vi "S2C_ExeScriptAbort.vi"(8 "Error In":errorcluster, 11 "Q-Ref":refnum<queue>) -> (0 "Error Out":errorcluster)   [LabVIEW 2015]
doc: "Changes the testing status to Aborted and calls the results case."
uses:
  Controls/S2C_ResultStatus.ctl
  Controls/S2C_ExePause.ctl
  Globals/S2C_Globals.vi
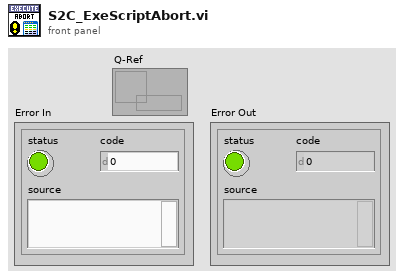
[diagram p1: front panel]
types:
  T1 = typedef "S2C_ExePause.ctl" = bool
  T2 = typedef "S2C_ResultStatus.ctl" = enum16{"Passed", "Failed", "Logged", "Aborted", "Error", "Testing...", "Paused", "No Record"}
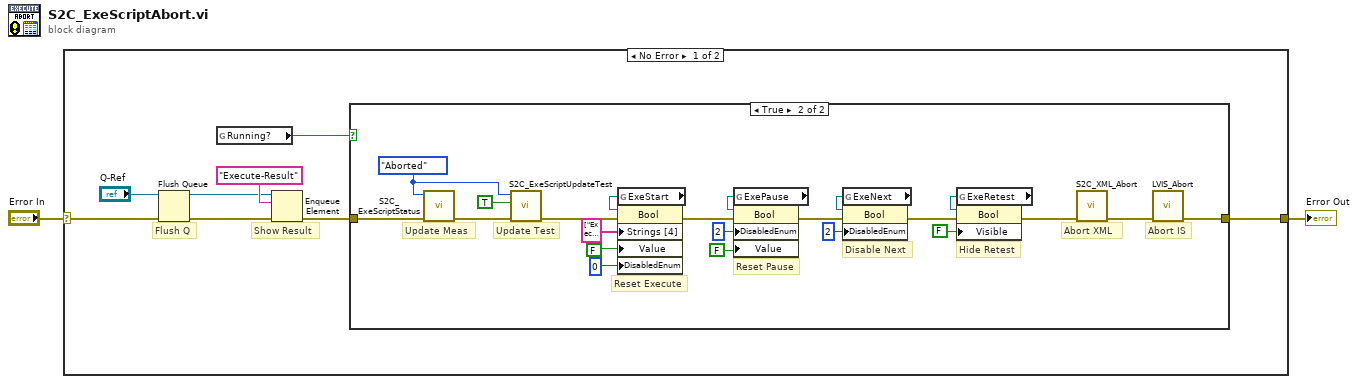
[diagram p0: block diagram]
diagram:
  n1 = case shown="No Error" "Error In" {
    selector: "Error In" -> [w8 w34]
    tunnel: [w7 w34] -> w1
    frame No Error {
      # "Show Result"
      # "Flush Q"
      n2 = Flush Queue(queue="Q-Ref", error in (no error)=w8) -> (queue out=w5:refnum<queue>, error out=w4:errorcluster)  [unwired: 1 out]
      n3 = global read "S2C_Globals.vi" "Running?"() -> (w10:bool)
      n4 = Enqueue Element(queue=w5, element="Execute-Result", error in (no error)=w4) -> (error out=w3:errorcluster)  [unwired: 1 in, 2 out]
      n5 = case shown="True" w10 {
        tunnel: [w11 w26] -> w7
        tunnel: w3 -> [w11 w33]
        frame False {
        }
        frame True {
          w18 = S2C_ResultStatus."Aborted" ("Status")
          # "Hide Retest"
          # "Update Test"
          # "Abort XML"
          # "Reset Execute"
          # "Abort IS"
          # "Disable Next"
          # "Reset Pause"
          # "Update Meas"
          n6 = call "S2C_ExeScriptStatus.vi"("Error In"=w33, "Status"=w18) -> ("Error Out"=w19:errorcluster)  [unwired: 9 in]
          n7 = call "S2C_ExeScriptUpdateTest.vi"("Error In"=w19, "LastMeas?"=TRUE, "Status"=w18) -> ("Error Out"=w17:errorcluster)  [unwired: 8 in]
          n8 = global read "S2C_Globals.vi" "ExeStart"() -> (w25:refnum<vi>)
          n9 = property on="Property Node" class="Bool"(reference=w25, error in=w17, "Strings [4]"=string[] ["Execute Script", "Abort Testing"] ("Array - String"), "Value"=T1 FALSE, "DisabledEnum"=u8 0) -> (error out=w22:errorcluster)  [unwired: 1 out]
          n10 = global read "S2C_Globals.vi" "ExePause"() -> (w32:refnum<vi>)
          n11 = property on="Property Node" class="Bool"(reference=w32, error in=w22, "DisabledEnum"=u8 2, "Value"=T1 FALSE) -> (error out=w28:errorcluster)  [unwired: 1 out]
          n12 = global read "S2C_Globals.vi" "ExeNext"() -> (w29:refnum<vi>)
          n13 = property on="Property Node" class="Bool"(reference=w29, error in=w28, "DisabledEnum"=u8 2) -> (error out=w15:errorcluster)  [unwired: 1 out]
          n14 = global read "S2C_Globals.vi" "ExeRetest"() -> (w16:refnum<vi>)
          n15 = property on="Property Node" class="Bool"(reference=w16, error in=w15, "Visible"=FALSE) -> (error out=w14:errorcluster)  [unwired: 1 out]
          n16 = call "S2C_XML_Abort.vi"("Error In"=w14) -> ("Error Out"=w20:errorcluster)  [unwired: 10 in]
          n17 = call "LVIS_Abort.vi"("Error In"=w20) -> ("Error Out"=w26:errorcluster)  [unwired: 10 in]
        }
      }
    }
    frame Error {
    }
  }
  "Error Out" <- w1
